vi "DB Info.vi"(8 "error in (no error)":errorcluster, 11 "MySQL in":refnum<class "MySQL.lvclass">) -> (0 "error out":errorcluster, 1 "Column_info":T1, 2 "Table_info":T4, 3 "MySQL out":refnum<class "MySQL.lvclass">)   [LabVIEW 2021, in "Database.lvlib" / "MySQL.lvclass"]
uses:
  MySQL.lvclass
  DB/Table_info.ctl
  DB/Column_info.ctl
  <vilib>/addons/database/Auxilliary.llb/DB Tools Column Info.ctl
  <vilib>/addons/database/Auxilliary.llb/DB Tools DataTypes.ctl
  DB/DB.lvclass
  <vilib>/addons/database/NI_Database_API.lvlib
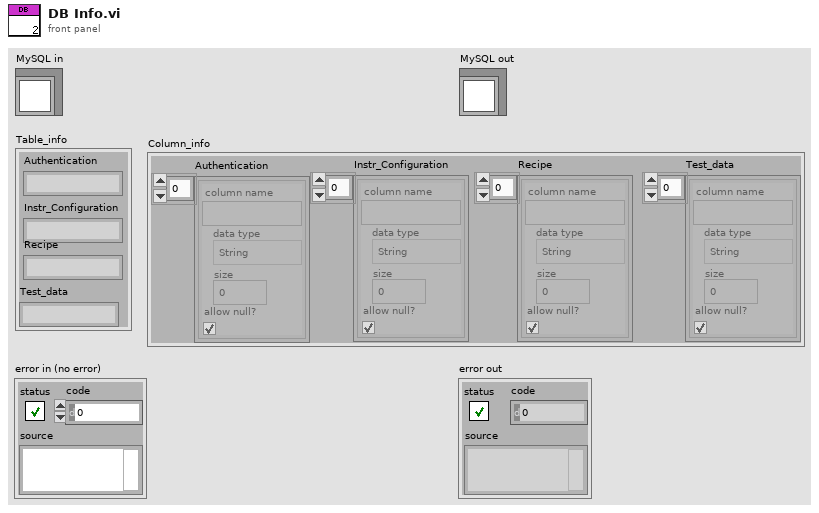
[diagram p1: front panel]
types:
  T1 = typedef "Database.lvlib/DB.lvclass/Column_info.ctl" = cluster{"Authentication":T2[], "Instr_Configuration":T2[], "Recipe":T2[], "Test_data":T2[]}
  T2 = typedef "NI_Database_API.lvlib/DB Tools Column Info.ctl" = cluster{"column name":string, "data type":T3, "size":i32, "allow null?":bool}
  T3 = typedef "NI_Database_API.lvlib/DB Tools DataTypes.ctl" = enum16{"String", "Long (I32)", "Single (SGL)", "Double (DBL)", "Date/Time", "Binary"}
  T4 = typedef "Database.lvlib/DB.lvclass/Table_info.ctl" = cluster{"Authentication":string, "Instr_Configuration":string, "Recipe":string, "Test_data":string}
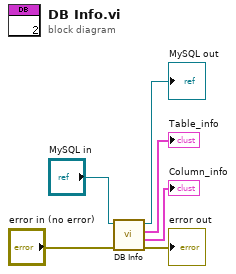
[diagram p0: block diagram]
diagram:
  n1 = call-parent "DB Info.vi"("error in (no error)"="error in (no error)", "DB in"="MySQL in") -> ("error out"=→"error out":errorcluster, "Column_info"=→"Column_info":T1, "Table_info"=→"Table_info":T4, "DB out"=→"MySQL out":refnum<class "MySQL.lvclass">)  [unwired: 6 in]
